vi "unloadSubVI.vi"(8 "error in":errorcluster, 11 "SubPanel in":refnum<class "xceSubPanel.lvclass">) -> (0 "error out":errorcluster, 2 "stoppedNode*":refnum<data-value>, 3 "SubPanel out":refnum<class "xceSubPanel.lvclass">)   [LabVIEW 2013, in "xceSubPanel.lvclass"]
doc: "Stops the current UI VI and removes the VI from the subpanel."
uses:
  xceSubPanel.lvclass
  xceDataNode/xceDataNode.lvclass
  xceSubPanel.lvclass/xceSubPanel.ctl
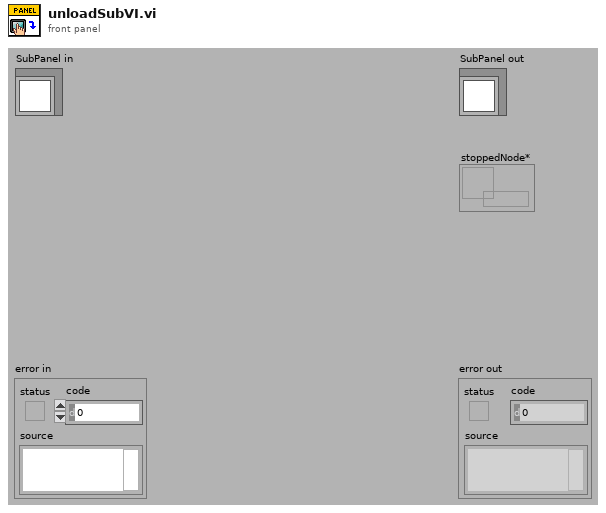
[diagram p1: front panel]
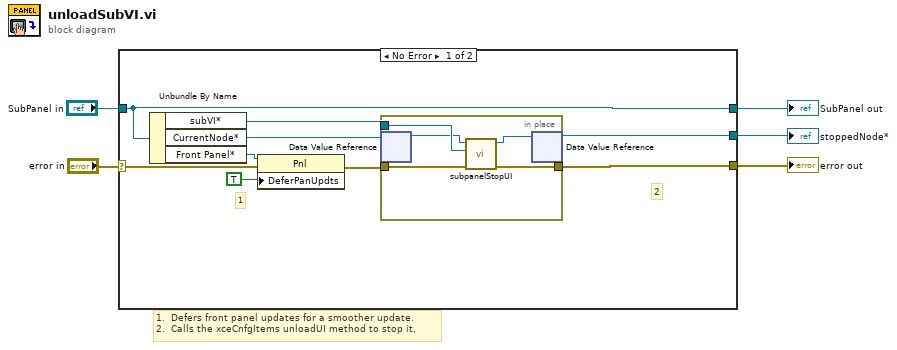
[diagram p0: block diagram]
diagram:
  # "1.  Defers front panel updates for a smoother update.\n2.  Calls the xceCnfgItems unloadUI method to stop it,"
  n1 = case shown="No Error" "error in" {
    selector: "error in" -> [w12 w21]
    tunnel: [w6 w21] -> w4
    tunnel: [w14 w20] -> w2
    tunnel: "SubPanel in" -> [w14 w20]
    tunnel: [w9 _] -> w1
    frame No Error {
      # "2"
      # "1"
      n2 = Unbundle By Name(w14) -> ("subVI*"=w8:refnum<vi>, "CurrentNode*"=w13:refnum<data-value>, "Front Panel*"=w11:refnum<vi>)
      n3 = property class="Pnl"(reference=w11, error in=w12, "DeferPanUpdts"=TRUE ("Defer Panel Updates")) -> (error out=w7:errorcluster)  [unwired: 1 out]
      n4 = in-place {
        in-place-border: w7 -> [w19]
        in-place-border: [w18] -> w6
        in-place-border: w8 -> [w16]
        n5 = in-place-dvr #1(w13) -> (w15:refnum<class "xceDataNode.lvclass">)  [unwired: 1 out]
        n6 = call "subpanelStopUI.vi"("error in (no error)"=w19, "UI VI*"=w16, "xceDataNode in"=w15) -> ("error out"=w18:errorcluster, "xceDataNode out"=w17:refnum<class "xceDataNode.lvclass">)  [unwired: 7 in]
        n7 = in-place-dvr #1(w17) -> (w9:refnum<data-value>)  [unwired: 1 out]
      }
    }
    frame Error {
    }
  }
  "error out" <- w4
  "SubPanel out" <- w2
  "stoppedNode*" <- w1
